vi "Default Instrument Setup.vi"(8 "error in (no error)":errorcluster, 11 "VISA resource name":refnum<visa-resource-name>) -> (0 "error out":errorcluster, 3 "VISA resource name out":refnum<visa-resource-name>)   [LabVIEW 2013, in "GP22_TDC_Arduinoed.lvlib"]
doc: "Sends a default command string to the instrument whenever a new VISA session is opened, or the instrument is reset. Use this VI as a subVI for the <b>Initialize</b> and <b>Reset</b> VIs. Altering this VI could cause these two VIs to operate incorrectly."
uses:
  GP22_TDC_Arduinoed.lvlib
  Public/Globals.vi
panel:
  out "Return message":string
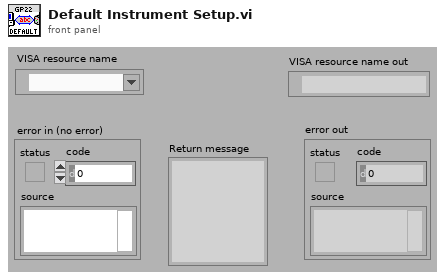
[diagram p1: front panel]
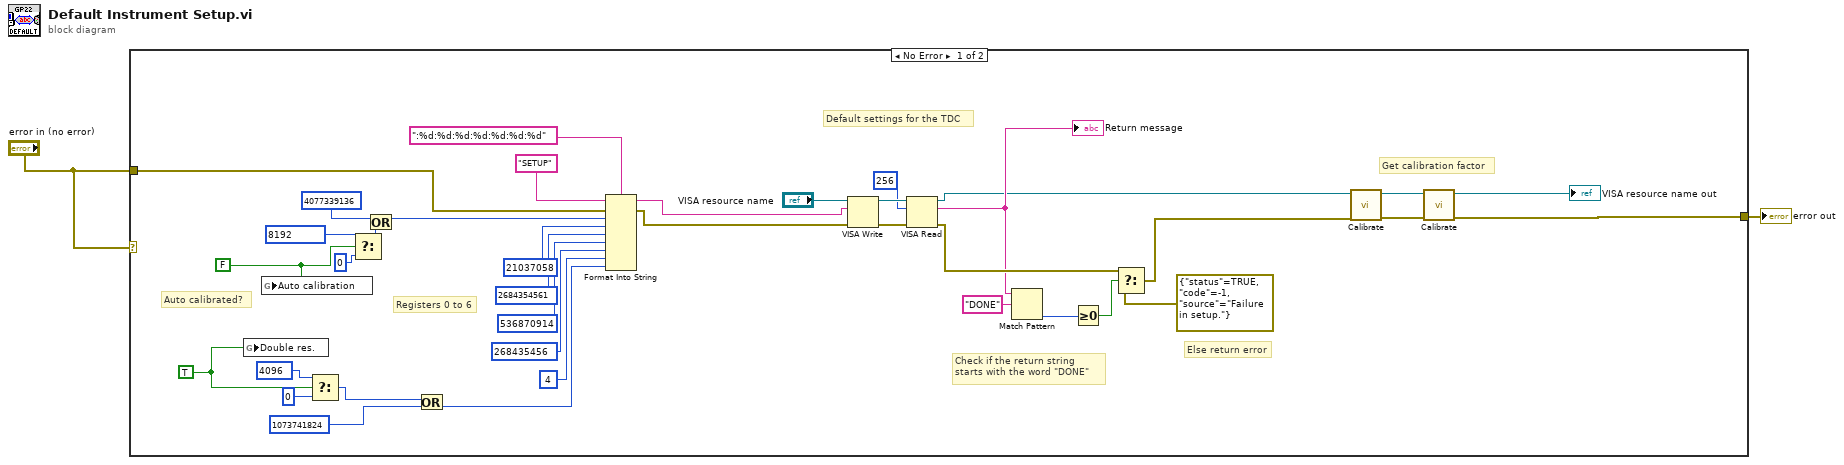
[diagram p0: block diagram]
diagram:
  n1 = case shown="No Error" "error in (no error)" {
    tunnel: "error in (no error)" -> [w29 w41]
    tunnel: [w9 w41] -> w2
    frame No Error {
      w6 = TRUE
      w15 = FALSE
      # "Get calibration factor"
      # "Auto calibrated?"
      # "Else return error"
      # "Check if the return string\nstarts with the word \"DONE\""
      # "Default settings for the TDC"
      # "Registers 0 to 6"
      n2 = global write "Globals.vi" "Double res."(w6) -> ()
      n3 = global write "Globals.vi" "Auto calibration"(w15) -> ()
      n4 = Select(t=u32 4096 ("input 1"), s=w6, f=u32 0) -> (s? t:f=w3:u32)
      n5 = Select(t=u32 8192 ("input 1"), s=w15, f=u32 0) -> (s? t:f=w18:u32)
      n6 = Or(x=u32 4077339136 ("input 1"), y=w18) -> (x .or. y?=w19:u32)
      n7 = Or(x=w3, y=u32 1073741824 ("input 1")) -> (x .or. y?=w7:u32)
      n8 = Format Into String(format string=":%d:%d:%d:%d:%d:%d:%d", initial string="SETUP", error in=w29, w19, u32 21037058 ("input 1"), u32 2684354561 ("input 1"), u32 536870914 ("input 1"), u32 268435456 ("input 1"), u32 4 ("input 1"), w7) -> (resulting string=w27:string, error out=w28:errorcluster)
      n9 = VISA Write(VISA resource name="VISA resource name", write buffer=w27, error in (no error)=w28) -> (VISA resource name out=w39:refnum<visa-resource-name>, error out=w26:errorcluster)  [unwired: 1 out]
      n10 = VISA Read(VISA resource name=w39, byte count=u32 256, error in (no error)=w26) -> (VISA resource name out=w13:refnum<visa-resource-name>, read buffer=w14:string, error out=w21:errorcluster)  [unwired: 1 out]
      "Return message" <- w14
      n11 = Match Pattern(string=w14, regular expression="DONE") -> (offset past match=w23:i32)  [unwired: 1 in, 3 out]
      n12 = Greater Or Equal To 0?(x=w23) -> (x >= 0?=w22:bool)
      n13 = Select(t=w21, s=w22, f=errorcluster {"status"=TRUE, "code"=-1, "source"="Failure in setup."}) -> (s? t:f=w12:errorcluster)
      n14 = call "Calibrate.vi"("error in (no error)"=w12, "VISA resource name"=w13) -> ("error out"=w10:errorcluster, "VISA resource name out"=w11:refnum<visa-resource-name>)  [unwired: 5 in, 2 out]
      n15 = call "Calibrate.vi"("error in (no error)"=w10, "VISA resource name"=w11) -> ("error out"=w9:errorcluster, "VISA resource name out"=→"VISA resource name out":refnum<visa-resource-name>)  [unwired: 5 in, 2 out]
    }
    frame Error {
    }
  }
  "error out" <- w2
